vi "Logic-CheckUpdateData.vi"(8 "error in (no error)":errorcluster, 11 "TableLogger Config":T1) -> (0 "error out":errorcluster, 3 "Update?T":bool)   [LabVIEW 2014, in "TableLogger_SQLite_Actor.lvlib" / "TableLogger_SQLite_Actor.lvclass"]
uses:
  TableLogger_SQLite_Actor.lvclass
  TableLogger_Actor/TableLoggerConfig.ctl
  TableLogger_Actor/TableLoggerTypes.ctl
  TableLogger_Actor/TableLoggerBackupConfig.ctl
  TableLogger_Actor/SelectConditionCriteria.ctl
  SelectConditions.ctl
  TableLogger_SQLite_Actor.lvclass/TableLogger_SQLite_Actor.ctl
  TableLogger_Actor/TableLogger_Actor.lvlib
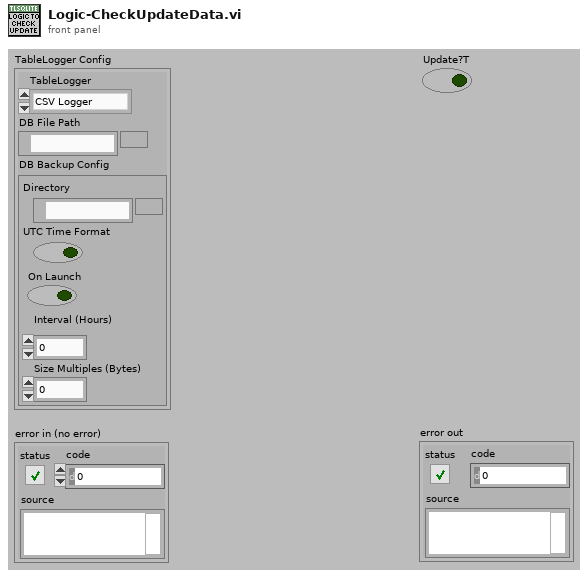
[diagram p1: front panel]
types:
  T1 = typedef "TableLogger_Actor.lvlib/TableLoggerConfig.ctl" = cluster{"TableLogger":T2, "DB File Path":path, "DB Backup Config":T3}
  T2 = typedef "TableLogger_Actor.lvlib/TableLoggerTypes.ctl" = enum16{"CSV Logger", "SQLite Logger"}
  T3 = typedef "TableLogger_Actor.lvlib/TableLoggerBackupConfig.ctl" = cluster{"Directory":path, "UTC Time Format":bool, "On Launch":bool, "Interval (Hours)":dbl, "Size Multiples (Bytes)":i32}
  T4 = typedef "TableLogger_Actor.lvlib/SelectConditionCriteria.ctl" = cluster{"Condition Data":variant[], "Recent N.Rows":string, "Select Type":T5}
  T5 = typedef "TableLogger_Actor.lvlib/SelectConditions.ctl" = enum16{"Select All", "AND Operator", "Recent Rows", "OR Operator", "BETWEEN Operator"}
  T6 = cluster{"Numeric Data":i32, "Float Data":dbl, "String Data":string, "Enum Data":enum16{"Enum Item 1", "Enum Item 2"}, "Array Data":i32[], "Array Data 2":i32[]}[]
  T7 = cluster{"Numeric Data":i32, "Float Data":dbl, "String Data":string, "Enum Data":enum16{"Enum Item 1", "Enum Item 2"}, "Array Data":i32[], "Array Data 2":i32[]}
  T8 = cluster{"Numeric Data":i32, "Float Data":dbl, "String Data":string, "Enum Data":enum16{"Enum Item 1", "Enum Item 2"}, "Array Data":i32[]}
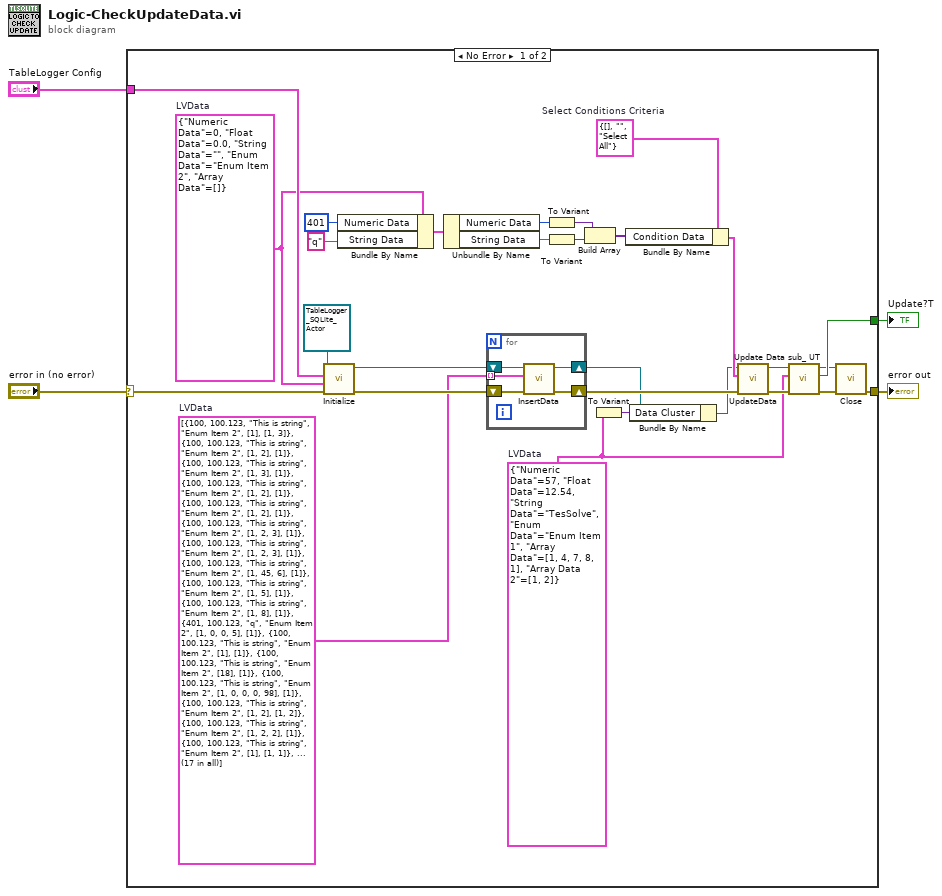
[diagram p0: block diagram]
diagram:
  n1 = case shown="No Error" "error in (no error)" {
    selector: "error in (no error)" -> [w30 w38]
    tunnel: [w21 w38] -> w4
    tunnel: "TableLogger Config" -> [w31 _]
    tunnel: [w29 _] -> w1
    frame No Error {
      w11 = T4 {"Condition Data"=[], "Recent N.Rows"="", "Select Type"=enum."Select All"}  # Select Conditions Criteria
      w24 = T6 [{"Numeric Data"=100, "Float Data"=100.123, "String Data"="This is string", "Enum Data"=enum."Enum Item 2", "Array Data"=[1], "Array Data 2"=[1, 3]}, {"Numeric Data"=100, "Float Data"=100.123, "String Data"="This is string", "Enum Data"=enum."Enum Item 2", "Array Data"=[1, 2], "Array Data 2"=[1]}, {"Numeric Data"=100, "Float Data"=100.123, "String Data"="This is string", "Enum Data"=enum."Enum Item 2", "Array Data"=[1, 3], "Array Data 2"=[1]}, {"Numeric Data"=100, "Float Data"=100.123, "String Data"="This is string", "Enum Data"=enum."Enum Item 2", "Array Data"=[1, 2], "Array Data 2"=[1]}, {"Numeric Data"=100, "Float Data"=100.123, "String Data"="This is string", "Enum Data"=enum."Enum Item 2", "Array Data"=[1, 2], "Array Data 2"=[1]}, {"Numeric Data"=100, "Float Data"=100.123, "String Data"="This is string", "Enum Data"=enum."Enum Item 2", "Array Data"=[1, 2, 3], "Array Data 2"=[1]}, {"Numeric Data"=100, "Float Data"=100.123, "String Data"="This is string", "Enum Data"=enum."Enum Item 2", "Array Data"=[1, 2, 3], "Array Data 2"=[1]}, {"Numeric Data"=100, "Float Data"=100.123, "String Data"="This is string", "Enum Data"=enum."Enum Item 2", "Array Data"=[1, 45, 6], "Array Data 2"=[1]}, {"Numeric Data"=100, "Float Data"=100.123, "String Data"="This is string", "Enum Data"=enum."Enum Item 2", "Array Data"=[1, 5], "Array Data 2"=[1]}, {"Numeric Data"=100, "Float Data"=100.123, "String Data"="This is string", "Enum Data"=enum."Enum Item 2", "Array Data"=[1, 8], "Array Data 2"=[1]}, {"Numeric Data"=401, "Float Data"=100.123, "String Data"="q", "Enum Data"=enum."Enum Item 2", "Array Data"=[1, 0, 0, 5], "Array Data 2"=[1]}, {"Numeric Data"=100, "Float Data"=100.123, "String Data"="This is string", "Enum Data"=enum."Enum Item 2", "Array Data"=[1], "Array Data 2"=[1]}, {"Numeric Data"=100, "Float Data"=100.123, "String Data"="This is string", "Enum Data"=enum."Enum Item 2", "Array Data"=[18], "Array Data 2"=[1]}, {"Numeric Data"=100, "Float Data"=100.123, "String Data"="This is string", "Enum Data"=enum."Enum Item 2", "Array Data"=[1, 0, 0, 0, 98], "Array Data 2"=[1]}, {"Numeric Data"=100, "Float Data"=100.123, "String Data"="This is string", "Enum Data"=enum."Enum Item 2", "Array Data"=[1, 2], "Array Data 2"=[1, 2]}, {"Numeric Data"=100, "Float Data"=100.123, "String Data"="This is string", "Enum Data"=enum."Enum Item 2", "Array Data"=[1, 2, 2], "Array Data 2"=[1]}, {"Numeric Data"=100, "Float Data"=100.123, "String Data"="This is string", "Enum Data"=enum."Enum Item 2", "Array Data"=[1], "Array Data 2"=[1, 1]}]  # LVData
      w9 = T7 {"Numeric Data"=57, "Float Data"=12.54, "String Data"="TesSolve", "Enum Data"=enum."Enum Item 1", "Array Data"=[1, 4, 7, 8, 1], "Array Data 2"=[1, 2]}  # LVData
      w12 = T8 {"Numeric Data"=0, "Float Data"=0.0, "String Data"="", "Enum Data"=enum."Enum Item 2", "Array Data"=[]}  # LVData
      n2 = call-dynamic "Initialize.vi"("error in (no error)"=w30, "Data Cluster (for Table Headers)"=w12, "TableLogger Config"=w31, "object in"=refnum<class "TableLogger_SQLite_Actor.lvclass"> refnum) -> ("error out"=w25:errorcluster, "object out"=w32:refnum<class "TableLogger_SQLite_Actor.lvclass">)  [unwired: 6 in]
      n3 = Bundle By Name(cluster=w12, "Numeric Data"=401, "String Data"="q") -> (w17:T8)
      n4 = Unbundle By Name(w17) -> ("Numeric Data"=w16:i32, "String Data"=w15:string)
      n5 = for {
        shift-right: [w36] -> w26
        shift-left: w25 -> [w37]
        shift-right: [w34] -> w7
        shift-left: w32 -> [w35]
        tunnel: w24 -> [w33] mode=indexing
        n6 = call-dynamic "InsertData.vi"("error in (no error)"=w37, "Data Cluster"=w33, "object in"=w35) -> ("error out"=w36:errorcluster, "object out"=w34:refnum<class "TableLogger_SQLite_Actor.lvclass">)  [unwired: 7 in]
      }
      n7 = To Variant(anything=w16) -> (Variant=w19:variant)
      n8 = To Variant(anything=w15) -> (Variant=w18:variant)
      n9 = Build Array(w19, w18) -> (w10:variant[])
      n10 = To Variant(anything=w9) -> (Variant=w5:variant)
      n11 = Bundle By Name(cluster=w11, "Condition Data"=w10) -> (w8:T4)
      n12 = Bundle By Name(cluster=w7, "Data Cluster"=w5) -> (w6:refnum<class "TableLogger_SQLite_Actor.lvclass">)
      n13 = call-dynamic "UpdateData.vi"("error in (no error)"=w26, "Select Conditions Criteria"=w8, "object in"=w6) -> ("error out"=w27:errorcluster, "object out"=w28:refnum<class "TableLogger_SQLite_Actor.lvclass">)  [unwired: 6 in, 1 out]
      n14 = call "Update Data sub_ UT.vi"("error in (no error)"=w27, "LVData"=w9, "TableLogger_SQLite_Actor in"=w28) -> ("error out"=w22:errorcluster, "Update?T"=w29:bool, "TableLogger_SQLite_Actor out"=w20:refnum<class "TableLogger_SQLite_Actor.lvclass">)  [unwired: 6 in]
      n15 = call-dynamic "Close.vi"("error in (no error)"=w22, "object in"=w20) -> ("error out"=w21:errorcluster)  [unwired: 8 in, 1 out]
    }
    frame Error {
    }
  }
  "error out" <- w4
  "Update?T" <- w1
